vi "Update Scale Label.vi"(8 "error in (no error)":errorcluster, 9 "y label":string, 10 "x label":string, 11 "[V] Waveform in":refnum<class "[V] Waveform.lvclass">) -> (0 "error out":errorcluster, 3 "[V] Waveform out":refnum<class "[V] Waveform.lvclass">)   [LabVIEW 2020, in "[V] Waveform.lvlib" / "[V] Waveform.lvclass"]
uses:
  [V] Waveform.lvclass
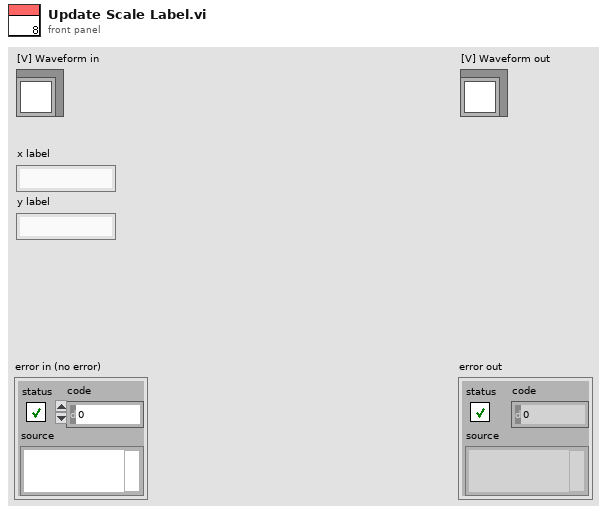
[diagram p1: front panel]
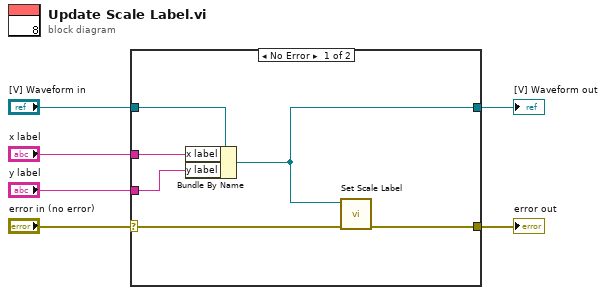
[diagram p0: block diagram]
diagram:
  n1 = case shown="No Error" "error in (no error)" {
    selector: "error in (no error)" -> [w12 w14]
    tunnel: [w11 w14] -> w5
    tunnel: [w7 w13] -> w3
    tunnel: "[V] Waveform in" -> [w10 w13]
    tunnel: "x label" -> [w9 _]
    tunnel: "y label" -> [w8 _]
    frame No Error {
      n2 = Bundle By Name(cluster=w10, "x label"=w9, "y label"=w8) -> (w7:refnum<class "[V] Waveform.lvclass">)
      n3 = call "Set Scale Label.vi"("error in (no error)"=w12, "[V] Waveform in"=w7) -> ("error out"=w11:errorcluster)  [unwired: 8 in, 1 out]
    }
    frame Error {
    }
  }
  "error out" <- w5
  "[V] Waveform out" <- w3
